vi "move_tilt_stage(Sub VI).vi"(0 "Axis inputs":T1={"Relative Steps"=0, "Motor Number"=1, "Run?"=FALSE, "Filename"=path "position.lvm", "CmdLib In"=refnum, "Device Address In"=0, "DeviceKey In"=""}, 1 "stop":bool, 2 "error in (no error)":errorcluster) -> (3 "CmdLib Out":refnum<k24>, 4 "DeviceKey Out":string, 5 "Position Status":i32, 6 "error out":errorcluster)   [LabVIEW 2016]
uses:
  C:/Users/UsphereLab/Documents/GitHub/Optlev/LabView Code/Tilt Stage/CmdLib.dll
  Tilt Stage/CmdLib.dll
panel:
  out "Description":string
  out "EOF?":bool
  out "Saving Data":bool
  out "Filename Out":path
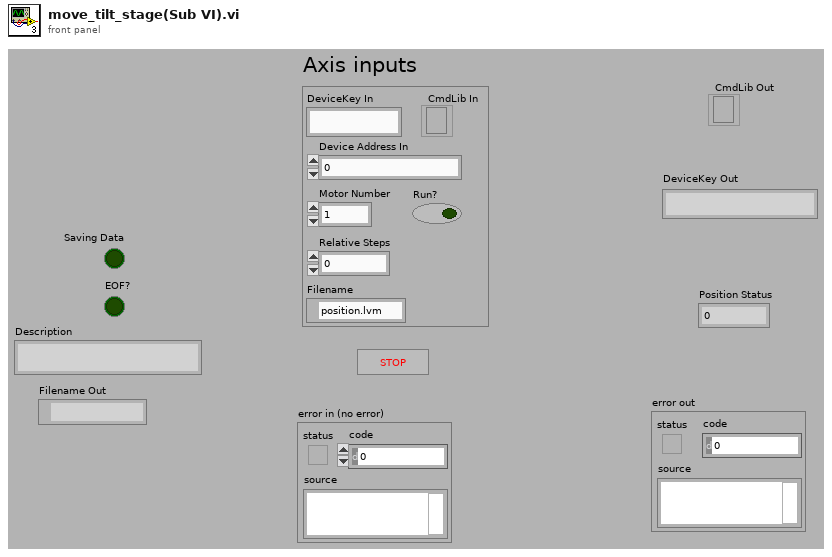
[diagram p1: front panel]
types:
  T1 = cluster{"Relative Steps":i32, "Motor Number":i32, "Run?":bool, "Filename":path, "CmdLib In":refnum<k24>, "Device Address In":i32, "DeviceKey In":string}
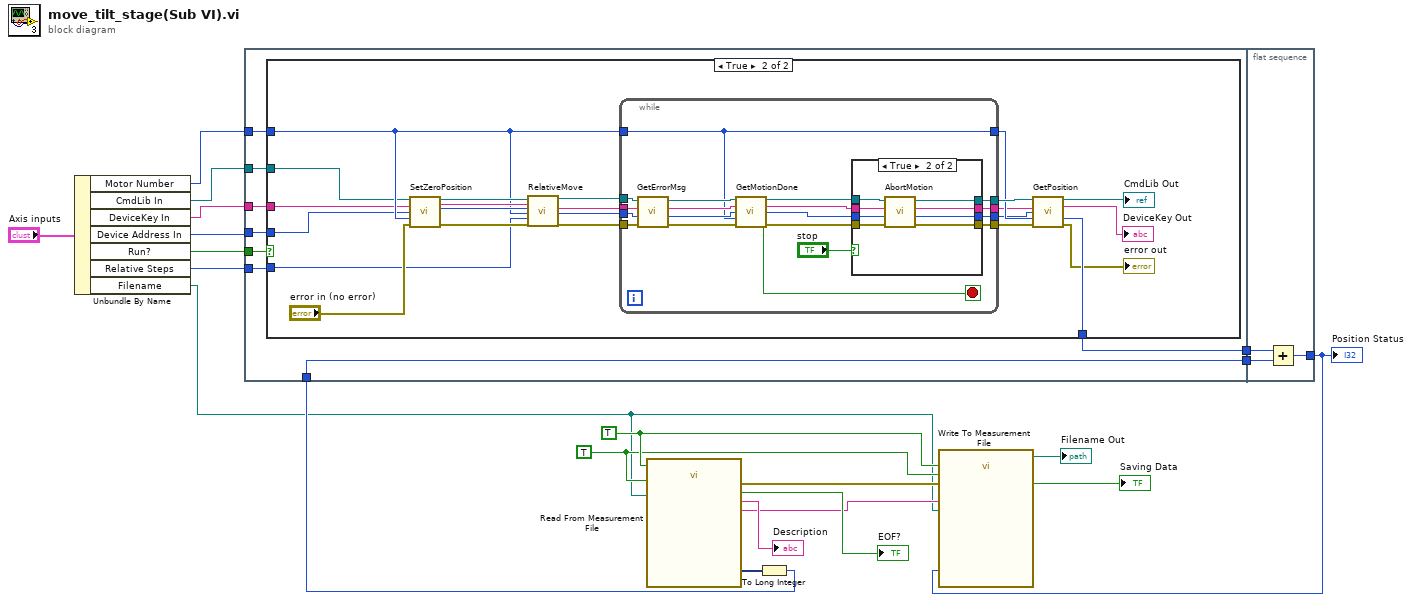
[diagram p0: block diagram]
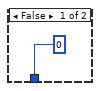
[diagram p2: hidden frame]
diagram:
  w11 = TRUE ("Enable")
  w12 = TRUE ("Reset")
  n1 = Unbundle By Name("Axis inputs") -> ("Motor Number"=w7:i32, "CmdLib In"=w6:refnum<k24>, "DeviceKey In"=w5:string, "Device Address In"=w4:i32, "Run?"=w3:bool, "Relative Steps"=w2:i32, "Filename"=w1:path)
  n2 = flat-sequence {
    tunnel: [w28] -> w21
    tunnel: w9 -> [w29]
    tunnel: [w29] -> w20
    tunnel: w7 -> [w27]
    tunnel: w6 -> [w26]
    tunnel: w5 -> [w25]
    tunnel: w4 -> [w24]
    tunnel: w3 -> [w23]
    tunnel: w2 -> [w22]
    tunnel: [w85] -> w19
    tunnel: w21 -> [w86]
    tunnel: w20 -> [w87]
    frame #0 {
      n3 = case shown="True" w23 {
        tunnel: [0 ("Relative Steps") w40] -> w28
        tunnel: w27 -> [_ w38]
        tunnel: w26 -> [_ w37]
        tunnel: w25 -> [_ w36]
        tunnel: w24 -> [_ w35]
        tunnel: w22 -> [_ w34]
        frame False {
        }
        frame True {
          n4 = call "SetZeroPosition.vi"("CmdLib In"=w37, "DeviceKey In"=w36, "Device Address In"=w35, "Motor"=w38, "error in (no error)"="error in (no error)") -> ("CmdLib Out"=w50:refnum<k24>, "DeviceKey Out"=w49:string, "Device Address Out"=w47:i32, "error out"=w48:errorcluster)  [unwired: 7 in]
          n5 = call "RelativeMove.vi"("CmdLib In"=w50, "DeviceKey In"=w49, "Device Address In"=w47, "Motor"=w38, "Relative Steps"=w34, "error in (no error)"=w48) -> ("CmdLib Out"=w53:refnum<k24>, "DeviceKey Out"=w52:string, "Device Address Out"=w46:i32, "error out"=w51:errorcluster)  [unwired: 10 in]
          n6 = while {
            tunnel: w38 -> [w57]
            tunnel: w53 -> [w70]
            tunnel: w52 -> [w69]
            tunnel: [w65] -> w44
            tunnel: w46 -> [w64]
            tunnel: w51 -> [w68]
            tunnel: [w66] -> w45
            tunnel: [w57] -> w43
            tunnel: [w56] -> w42
            tunnel: [w55] -> w41
            stop <- w62 stop-if-true
            n7 = call "GetErrorMsg.vi"("error in (no error)"=w68, "Device Address In"=w64, "DeviceKey In"=w69, "CmdLib In"=w70) -> ("error out"=w67:errorcluster, "Device Address Out"=w63:i32, "DeviceKey Out"=w72:string, "CmdLib Out"=w71:refnum<k24>)
            n8 = call "GetMotionDone.vi"("CmdLib In"=w71, "DeviceKey In"=w72, "Device Address In"=w63, "Motor"=w57, "error in (no error)"=w67) -> ("CmdLib Out"=w61:refnum<k24>, "DeviceKey Out"=w60:string, "Device Address Out"=w59:i32, "Is Motion Done"=w62:bool, "error out"=w58:errorcluster)  [unwired: 6 in]
            n9 = case shown="True" "stop" {
              tunnel: w58 -> [w75 w84]
              tunnel: [w75 w83] -> w66
              tunnel: w61 -> [w76 w82]
              tunnel: [w76 w81] -> w65
              tunnel: w60 -> [w73 w80]
              tunnel: w59 -> [w74 w79]
              tunnel: [w74 w78] -> w56
              tunnel: [w73 w77] -> w55
              frame False {
              }
              frame True {
                n10 = call "AbortMotion.vi"("error in (no error)"=w84, "Device Address In"=w79, "DeviceKey In"=w80, "CmdLib In"=w82) -> ("error out"=w83:errorcluster, "Device Address Out"=w78:i32, "DeviceKey Out"=w77:string, "CmdLib Out"=w81:refnum<k24>)
              }
            }
          }
          n11 = call "GetPosition.vi"("CmdLib In"=w44, "DeviceKey In"=w41, "Device Address In"=w42, "Motor"=w43, "error in (no error)"=w45) -> ("CmdLib Out"=→"CmdLib Out":refnum<k24>, "DeviceKey Out"=→"DeviceKey Out":string, "Position"=w40:i32, "error out"=→"error out":errorcluster)  [unwired: 6 in, 1 out]
        }
      }
    }
    frame #1 {
      n12 = Add(x=w86, y=w87) -> (x+y=w85:i32)
    }
  }
  n13 = call "Read From Measurement File"("Filename"=w1, "Enable"=w11, "Reset"=w12) -> ("error out"=w14:errorcluster, "Signals"=w10:dynamicdata, "EOF?"=→"EOF?":bool, "Comment"=w13:string, "Description"=→"Description":string)  [unwired: 3 in, 1 out]
  n14 = To Long Integer(number=w10) -> (32bit integer=w9:i32)
  n15 = call "Write To Measurement File"("Signals"=w19, "Reset"=w12, "Enable"=w11, "error in (no error)"=w14, "Filename"=w1, "Comment"=w13) -> ("Filename Out"=→"Filename Out":path, "Saving Data"=→"Saving Data":bool)  [unwired: 11 in, 1 out]
  "Position Status" <- w19
